vi "window_graph calc_area.vi"(0 "baseline data":cluster{"X":dbl, "Y":dbl}[](array[cluster]), 1 "vaild region data":cluster{"X":dbl, "Y":dbl}[](array[cluster])) -> (2 "area":dbl, 3 "height":dbl, 4 "half-height width":dbl)   [LabVIEW 2018]
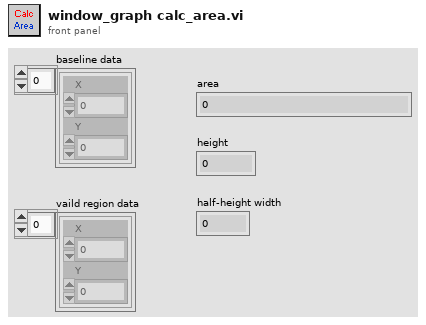
[diagram p1: front panel]
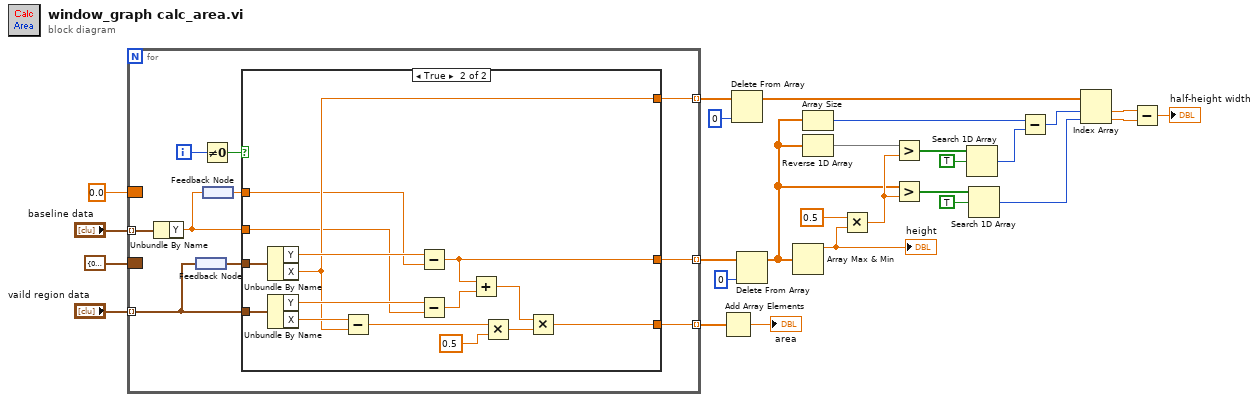
[diagram p0: block diagram]
diagram:
  n1 = for {
    tunnel: "baseline data" -> [w30] mode=indexing
    tunnel: "vaild region data" -> [w35] mode=indexing
    border: cluster{"X":dbl, "Y":dbl} {"X"=0.0, "Y"=0.0} ("mouse down pos") -> [_]
    tunnel: [w33] -> w24 mode=indexing
    tunnel: [w32] -> w22 mode=indexing
    tunnel: [w31] -> w7 mode=indexing
    border: 0.0 ("Y") -> [_]
    i -> [w37]
    n2 = Unbundle By Name(w30) -> ("Y"=w29:dbl)
    n3 = feedback #1() -> (w34:cluster{"X":dbl, "Y":dbl})
    n4 = feedback-in #1(w35) -> ()
    n5 = Not Equal To 0?(x=w37) -> (x != 0?=w36:bool)
    n6 = feedback #2() -> (w28:dbl)
    n7 = feedback-in #2(w29) -> ()
    n8 = case shown="True" w36 {
      tunnel: w35 -> [_ w51]
      tunnel: w34 -> [_ w52]
      tunnel: [_ w43] -> w33
      tunnel: [_ w41] -> w32
      tunnel: [_ w40] -> w31
      tunnel: w29 -> [_ w38]
      tunnel: w28 -> [_ w39]
      frame False {
      }
      frame True {
        n9 = Unbundle By Name(w52) -> ("Y"=w50:dbl, "X"=w40:dbl)
        n10 = Unbundle By Name(w51) -> ("Y"=w42:dbl, "X"=w49:dbl)
        n11 = Subtract(x=w49, y=w40) -> (x-y=w47:dbl)
        n12 = Subtract(x=w50, y=w39) -> (x-y=w41:dbl)
        n13 = Subtract(x=w42, y=w38) -> (x-y=w48:dbl)
        n14 = Add(x=w41, y=w48) -> (x+y=w45:dbl)
        n15 = Multiply(x=w47, y=0.5) -> (x*y=w44:dbl)
        n16 = Multiply(x=w45, y=w44) -> (x*y=w43:dbl)
      }
    }
  }
  n17 = Add Array Elements(numeric array=w24) -> (sum=→"area":dbl)
  n18 = Delete From Array(array=w7, index=0) -> (array with subset deleted=w6:dbl[])  [unwired: 1 in, 1 out]
  n19 = Delete From Array(array=w22, index=0) -> (array with subset deleted=w5:dbl[])  [unwired: 1 in, 1 out]
  n20 = Array Max & Min(array=w5) -> (max value=w12:dbl)  [unwired: 3 out]
  "height" <- w12
  n21 = Array Size(array=w5) -> (size(s)=w4:i32)
  n22 = Reverse 1D Array(array=w5) -> (reversed array=w9:dbl[])
  n23 = Multiply(x=0.5 ("y"), y=w12) -> (x*y=w16:dbl)
  n24 = Greater?(x=w9, y=w16) -> (0:w19:bool[])
  n25 = Greater?(x=w5, y=w16) -> (0:w18:bool[])
  n26 = Search 1D Array(1D array=w19, element=TRUE) -> (index of element=w3:i32)  [unwired: 1 in]
  n27 = Search 1D Array(1D array=w18, element=TRUE) -> (index of element=w15:i32)  [unwired: 1 in]
  n28 = Subtract(x=w4, y=w3) -> (x-y=w2:i32)
  n29 = Index Array(array=w6, index #1=w2, index #2=w15) -> (element #1=w10:dbl, element #2=w14:dbl)
  n30 = Subtract(x=w10, y=w14) -> (x-y=→"half-height width":dbl)
